vi "String.Remove Start and End Quotes.vi"(8 "error in":errorcluster, 11 "String In":string) -> (0 "error out":errorcluster, 3 "String Out":string)   [LabVIEW 2024, in "EQMF.lvlib" / "String Utils.lvlib"]
uses:
  String Utils.lvlib
  <vilib>/Utility/error.llb/Trim Whitespace One-Sided.vi
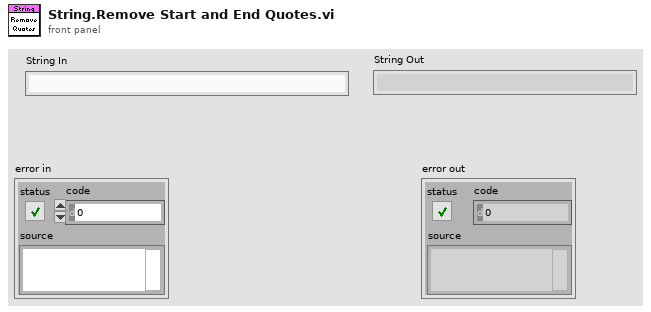
[diagram p1: front panel]
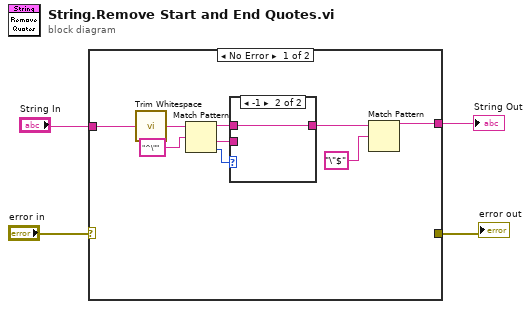
[diagram p0: block diagram]
diagram:
  n1 = case shown="No Error" "error in" {
    selector: "error in" -> [_ w17]
    tunnel: [w6 w16] -> w4
    tunnel: "String In" -> [w5 w16]
    tunnel: [_ w17] -> w1
    frame No Error {
      n2 = call <vilib>:"Trim Whitespace.vi"("string"=w5) -> ("trimmed string"=w13:string)  [unwired: 1 in]
      n3 = Match Pattern(string=w13, regular expression="^\"" ("replace string (\"\")")) -> (before substring=w10:string, after substring=w9:string, offset past match=w11:i32)  [unwired: 1 in, 1 out]
      n4 = case shown="-1" w11 {
        tunnel: w10 -> [_ w15]
        tunnel: w9 -> [w14 _]
        tunnel: [w14 w15] -> w8
        frame 0, Default {
        }
        frame -1 {
        }
      }
      n5 = Match Pattern(string=w8, regular expression="\"$" ("replace string (\"\")")) -> (before substring=w6:string)  [unwired: 1 in, 3 out]
    }
    frame Error {
    }
  }
  "String Out" <- w4
  "error out" <- w1
